vi "Get Producer Values.vi"(8 "error in":errorcluster, 11 "Device Cluster.lvclass":refnum<class "Device Cluster.lvclass">) -> (0 "error out":errorcluster, 2 "Producer Ch":cluster{"Voltage.AV":dbl, "Current.AV":dbl}[](array[cluster]), 3 "Device Cluster.lvclass out":refnum<class "Device Cluster.lvclass">)   [LabVIEW 2023, in "Device Cluster.lvclass"]
uses:
  Device Cluster.lvclass
  Device Cluster.lvclass/Device Cluster.ctl
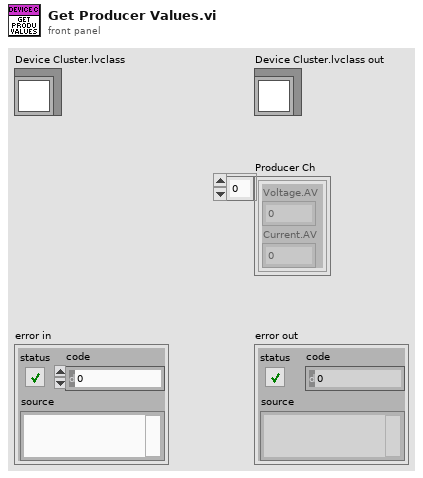
[diagram p1: front panel]
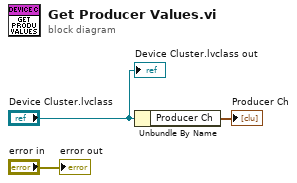
[diagram p0: block diagram]
diagram:
  n1 = Unbundle By Name("Device Cluster.lvclass") -> ("Producer Ch"=→"Producer Ch":cluster{"Voltage.AV":dbl, "Current.AV":dbl}[])
  "Device Cluster.lvclass out" <- "Device Cluster.lvclass"
  "error out" <- "error in"
